vi "Select VI Ref.vi"(8 "error in (no error)":errorcluster, 10 "Module Name":string, 11 "All Module Ref":refnum<vi>[](array[refnum])) -> (0 "error out":errorcluster, 2 "VI Refnum":refnum<vi>)   [LabVIEW 2020]
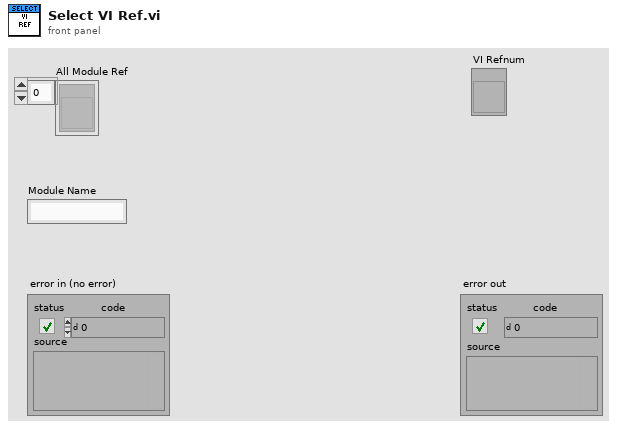
[diagram p1: front panel]
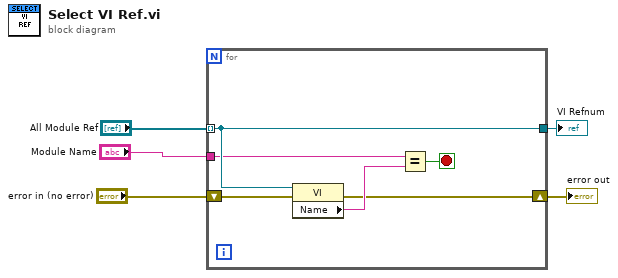
[diagram p0: block diagram]
diagram:
  n1 = for {
    tunnel: "Module Name" -> [w7]
    tunnel: "All Module Ref" -> [w9] mode=indexing
    tunnel: [w9] -> w1
    shift-right: [w8] -> w2
    shift-left: "error in (no error)" -> [w11]
    stop <- w6 stop-if-true
    n2 = property class="VI"(reference=w9, error in=w11) -> (error out=w8:errorcluster, "Name"=w10:string)  [unwired: 1 out]
    n3 = Equal?(x=w7, y=w10) -> (x = y?=w6:bool)
  }
  "error out" <- w2
  "VI Refnum" <- w1
